vi "UpdateVarFromJSON.vi"(8 "error in (no error)":errorcluster, 10 "JSON Variable Object":string, 11 "Variable.lvclass":refnum<class "Variable.lvclass">) -> (0 "error out":errorcluster, 3 "reference out":refnum<class "Variable.lvclass">)   [LabVIEW 2013]
doc: "Takes the passed JSON representation of the variable and applies the value to the passed in variable, interpreting 'null' in the JSON as leaving the value unchanged."
uses:
  VariableManagerCodes/Variable/Variable.lvclass
  JSONVariable.ctl
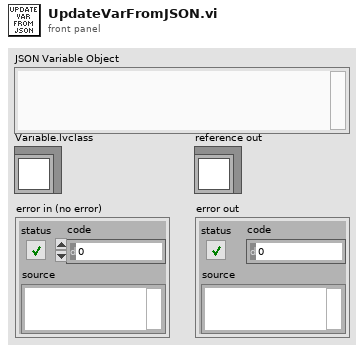
[diagram p1: front panel]
types:
  T1 = typedef "JSONVariable.ctl" = cluster{"name":string, "defaultValue":dbl, "sequenceFunction":string, "informIgor":bool, "sequence":bool}
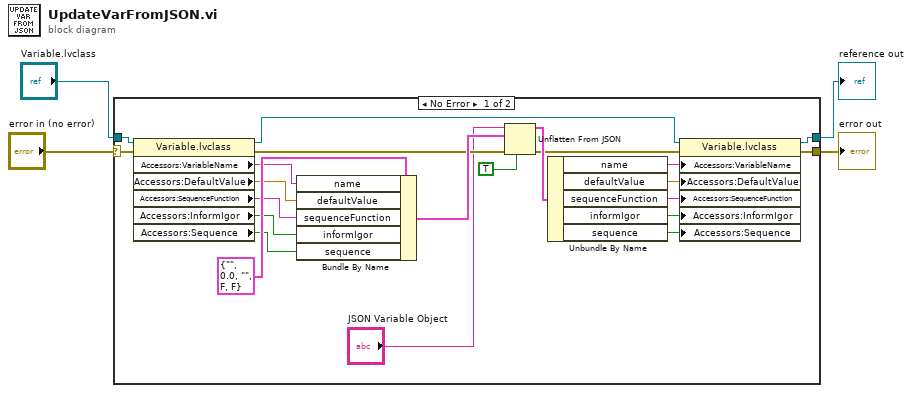
[diagram p0: block diagram]
diagram:
  n1 = case shown="No Error" "error in (no error)" {
    selector: "error in (no error)" -> [w5 w27]
    tunnel: "Variable.lvclass" -> [w26 w28]
    tunnel: [w7 w28] -> w3
    tunnel: [w6 w27] -> w2
    frame No Error {
      n2 = property class="Variable.lvclass"(reference=w26, error in=w5) -> (reference out=w16:refnum<class "Variable.lvclass">, error out=w15:errorcluster, "Accessors:VariableName"=w24:string, "Accessors:DefaultValue"=w23:dbl, "Accessors:SequenceFunction"=w22:string, "Accessors:InformIgor"=w21:bool, "Accessors:Sequence"=w20:bool)
      n3 = Bundle By Name(cluster=T1 {"name"="", "defaultValue"=0.0, "sequenceFunction"="", "informIgor"=FALSE, "sequence"=FALSE} ("JSONVariable"), "name"=w24, "defaultValue"=w23, "sequenceFunction"=w22, "informIgor"=w21, "sequence"=w20) -> (w19:T1)
      n4 = Unflatten From JSON(JSON string="JSON Variable Object", type and defaults=w19, default null elements? (F)=TRUE, error in (no error)=w15) -> (value=w17:T1, error out=w14:errorcluster)  [unwired: 3 in]
      n5 = Unbundle By Name(w17) -> ("name"=w13:string, "defaultValue"=w12:dbl, "sequenceFunction"=w11:string, "informIgor"=w10:bool, "sequence"=w9:bool)
      n6 = property class="Variable.lvclass"(reference=w16, error in=w14, "Accessors:VariableName"=w13, "Accessors:DefaultValue"=w12, "Accessors:SequenceFunction"=w11, "Accessors:InformIgor"=w10, "Accessors:Sequence"=w9) -> (reference out=w7:refnum<class "Variable.lvclass">, error out=w6:errorcluster)
    }
    frame Error {
    }
  }
  "reference out" <- w3
  "error out" <- w2
